vi "Constants.vi"() -> ()   [LabVIEW 2016, in "VeriStand Configuration Support.lvlib"]
uses:
  VeriStand Configuration Support.lvlib
panel:
  in  "Mediator Settings":string="Mediator.Settings"
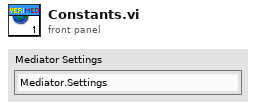
[diagram p1: front panel]
diagram:
